vi "abouttest - Copy.vi"   [LabVIEW 2015]
uses:
  board.vis/Globals.vi
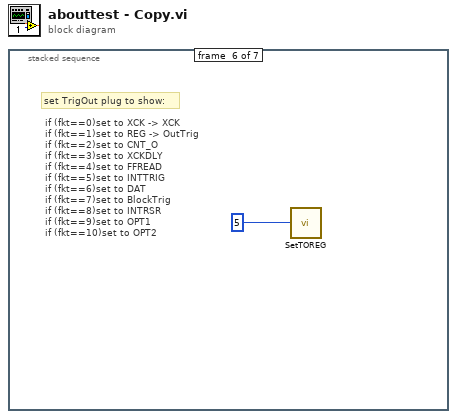
[diagram p0: block diagram]
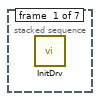
[diagram p2: hidden frame]
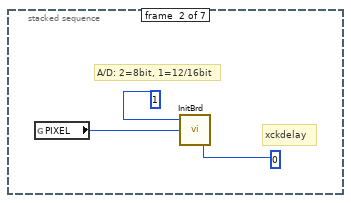
[diagram p3: hidden frame]
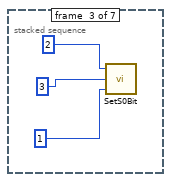
[diagram p4: hidden frame]
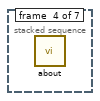
[diagram p5: hidden frame]
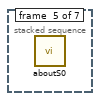
[diagram p6: hidden frame]
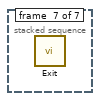
[diagram p7: hidden frame]
diagram:
  n1 = stacked-sequence {
    frame #0 {
      n2 = call "InitDrv.vi"() -> ()  [unwired: 1 in, 1 out]
    }
    frame #1 {
      # "xckdelay"
      # "A/D: 2=8bit, 1=12/16bit"
      n3 = global read "Globals.vi" "PIXEL"() -> (w1:u32)
      n4 = call "InitBrd.vi"("xckdly"=u32 0, "pixel"=w1, "flag816"=u32 1) -> ()  [unwired: 3 in]
    }
    frame #2 {
      n5 = call "SetS0Bit.vi"("drv"=u32 1, "Address"=u8 3, "bitnumber"=u32 2) -> ()
    }
    frame #3 {
      n6 = call "about.vi"() -> ()  [unwired: 2 in]
    }
    frame #4 {
      n7 = call "aboutS0.vi"() -> ()  [unwired: 1 in]
    }
    frame #5 {
      # "set TrigOut plug to show:"
      # "if (fkt==0)set to XCK -> XCK\nif (fkt==1)set to REG -> OutTrig\nif (fkt==2)set to CNT_O\nif (fkt==3)set to XCKDLY\nif (fkt==4)set to FFREAD\nif (fkt==5)set to INTTRIG\nif (fkt==6)set to DAT\nif (fkt==7)set to BlockTrig\nif (fkt==8)set to INTRSR\nif (fkt==9)set to OPT1\nif (fkt==10)set to OPT2"
      n8 = call "SetTOREG.vi"("fkt"=u8 5) -> ()
    }
    frame #6 {
      n9 = call "Exit.vi"() -> ()  [unwired: 1 in]
    }
  }
